vi "DifSignGenAdq_Activity3.vi"() -> ()   [LabVIEW 2015]
panel:
  in  "stop":bool
  out "Waveform Graph 3":dynamicdata(graph)
  out "Waveform Graph 2":dynamicdata(graph)
  out "Waveform Graph":dynamicdata(graph)
  in  "Standar":dbl(slide) caption="Offset" scale=0.0..10.0
  in  "Selector de\nSeñal":bool
  in  "Offset":dbl(slide) scale=0.0..10.0
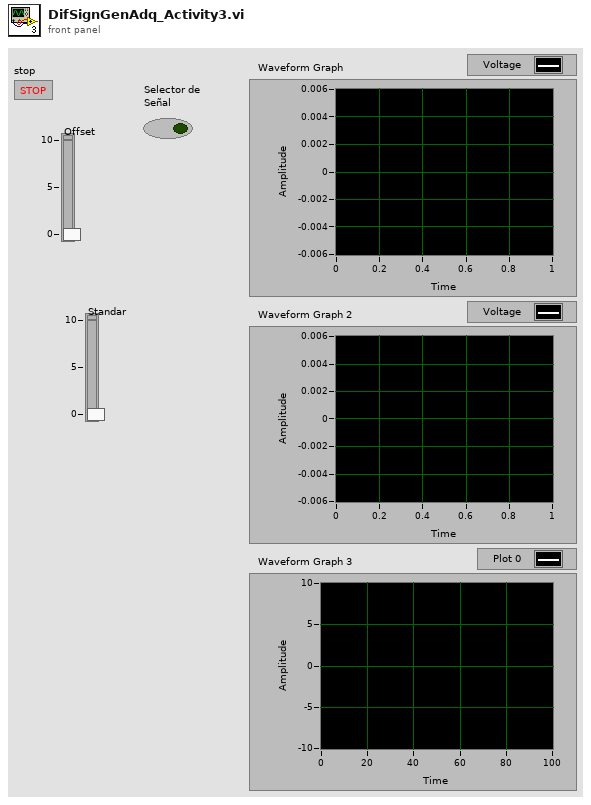
[diagram p1: front panel]
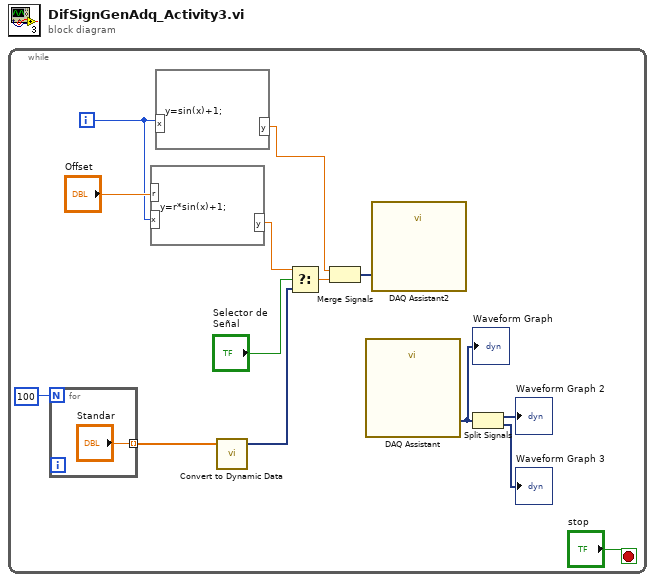
[diagram p0: block diagram]
diagram:
  n1 = while {
    i -> [w2]
    stop <- "stop" stop-if-true
    n2 = for {
      N: 100 -> [_]
      tunnel: ["Standar"] -> w11 mode=indexing
    }
    n3 = formula code="y=r*sin(x)+1;"("x"=w2, "r"="Offset") -> ("y"=w1:dbl)
    n4 = formula code="y=sin(x)+1;"("x"=w2) -> ("y"=w4:dbl)
    n5 = call "Convert to Dynamic Data"("Waveform"=w11) -> ("Dynamic Data Type"=w10:dynamicdata)  [unwired: 3 in]
    n6 = Select(t=w1, s="Selector de\nSeñal", f=w10) -> (s? t:f=w13:dbl)
    n7 = Merge Signals(w4, w13) -> (w9:dynamicdata)
    n8 = call "DAQ Assistant"() -> ("data"=w8:dynamicdata)  [unwired: 16 in, 3 out]
    "Waveform Graph" <- w8
    n9 = call "DAQ Assistant2"("data"=w9) -> ()  [unwired: 17 in, 2 out]
    n10 = Split Signals(w8) -> (→"Waveform Graph 2":dynamicdata, →"Waveform Graph 3":dynamicdata)  [unwired: 2 in]
  }
